vi "convertToKeyValuePair_2DArray.vi"(8 "error in (no error)":errorcluster, 9 "presicion (0)":u8, 10 "value":dbl[][](array[numeric])=[[1.2, 0.3]], 11 "name":string) -> (0 "error out":errorcluster, 3 "string converted":string)   [LabVIEW 2018]
doc: "Convert a 2-dimension array into a key value pair as string."
uses:
  convertToKeyValuePair_string.vi
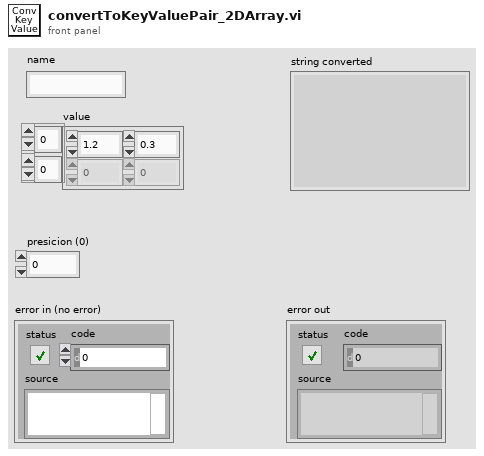
[diagram p1: front panel]
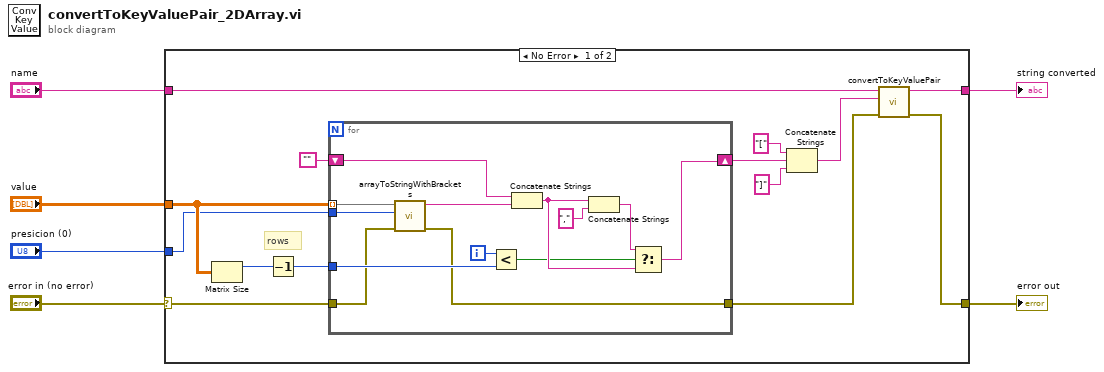
[diagram p0: block diagram]
diagram:
  n1 = case shown="No Error" "error in (no error)" {
    selector: "error in (no error)" -> [w12 w34]
    tunnel: [w10 _] -> w6
    tunnel: "name" -> [w11 _]
    tunnel: [w7 w34] -> w3
    tunnel: "value" -> [w18 _]
    tunnel: "presicion (0)" -> [w13 _]
    frame No Error {
      # "rows"
      n2 = Matrix Size(0:w18) -> (1:w17:i32)  [unwired: 1 out]
      n3 = Decrement(x=w17) -> (x-1=w16:i32)
      n4 = for {
        tunnel: w18 -> [w25] mode=indexing
        tunnel: w16 -> [w26]
        shift-right: [w28] -> w14
        shift-left: "" -> [w29]
        tunnel: w13 -> [w24]
        tunnel: w12 -> [w22]
        tunnel: [w21] -> w8
        i -> [w27]
        n5 = call "arrayToStringWithBrackets.vi"("error in (no error)"=w22, "presicion (0)"=w24, "value"=w25) -> ("error out"=w21:errorcluster, "String"=w23:string)  [unwired: 7 in]
        n6 = Less?(x=w27, y=w26) -> (x < y?=w31:bool)
        n7 = Concatenate Strings(w29, w23) -> (w33:string)
        n8 = Concatenate Strings(w33, ",") -> (w32:string)
        n9 = Select(t=w32, s=w31, f=w33) -> (s? t:f=w28:string)
      }
      n10 = Concatenate Strings("[" ("string"), w14, "]" ("string")) -> (w9:string)
      n11 = call-poly "convertToKeyValuePair.vi"("error in (no error)"=w8, "value"=w9, "name"=w11) -> ("error out"=w7:errorcluster, "string converted"=w10:string)  [unwired: 7 in]
    }
    frame Error {
    }
  }
  "error out" <- w3
  "string converted" <- w6
